vi "Edit Line.vi"(8 "error in (no error)":errorcluster, 10 "Line Name":string, 11 "object Refs":T1) -> (0 "error out":errorcluster, 1 "Change":bool)   [LabVIEW 2013, in "Modbus Module editor node.lvclass"]
uses:
  Modbus Module editor node.lvclass
  <vilib>/NI/DCAF/Tag Editor Core/Table API/Table Manager/object ref.ctl
  <vilib>/NI/DCAF/Tag Editor Core/Configuration Editor/Classes/Engine Parent/Engine Parent Editor Node.lvclass
  <vilib>/NI/DCAF/Tag Editor Core/Configuration Editor/Classes/Module editor node/module editor node.lvclass
  module/configuration/Modbus Module configuration.lvclass
  table line.ctl
  module/module channel/Modbus Module Channel.lvclass
  <vilib>/NI/Configuration Framework/serializable configuration/NISE_CEF_serializable configuration.lvclass/NISE_CEF_serializable configuration.ctl
  <vilib>/NI/Tag Bus/tag/tag descriptor.lvclass/tag descriptor.ctl
  <vilib>/Utility/LVClass/Get LV Class Name.vi
  <vilib>/NI/Configuration Framework/error generator/NISE_error generator.vi
  <vilib>/NI/Module Execution Interface/Engine Configuration/engine configuration.lvclass
  <vilib>/NI/Tag Bus/tag/tag descriptor.lvclass
  <vilib>/NI/Configuration Framework/serializable configuration/NISE_CEF_serializable configuration.lvclass
  <vilib>/NI/DCAF/Tag Editor Core/Table API/Table Manager/Table Manager.lvclass
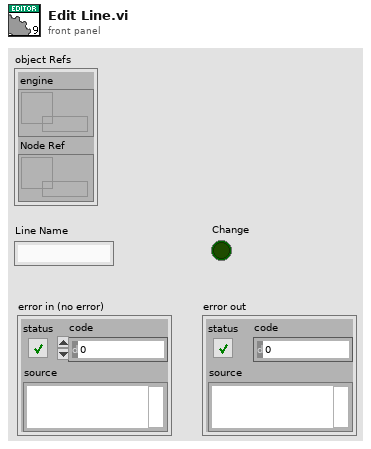
[diagram p1: front panel]
types:
  T1 = typedef "Table Manager.lvlib/Table Manager.lvclass/object ref.ctl" = cluster{"engine":refnum<data-value>, "Node Ref":refnum<data-value>}
  T2 = typedef "Modbus Module editor node.lvclass/table line.ctl" = cluster{"mbchan":refnum<class "Modbus Module Channel.lvclass">, "tag name":string}
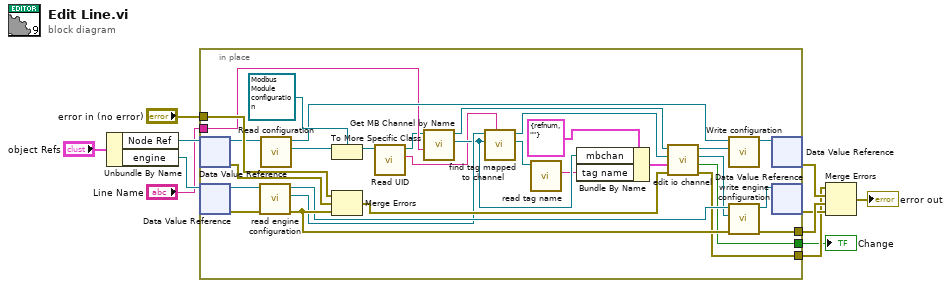
[diagram p0: block diagram]
diagram:
  n1 = Unbundle By Name("object Refs") -> ("Node Ref"=w4:refnum<data-value>, "engine"=w3:refnum<data-value>)
  n2 = in-place {
    in-place-border: [w33] -> w6
    in-place-border: "error in (no error)" -> [w41]
    in-place-border: [w35] -> w8
    in-place-border: "Line Name" -> [w22]
    in-place-border: [w12] -> w1
    n3 = in-place-dvr #1(w4) -> (w25:refnum<class "module editor node.lvclass">, w34:errorcluster)
    n4 = in-place-dvr #2(w3) -> (w40:refnum<class "Engine Parent Editor Node.lvclass">, w39:errorcluster)
    n5 = call <vilib>:"read engine configuration.vi"("error in"=w39, "Engine Parent Editor Node in"=w40) -> ("error out"=w37:errorcluster, "engine configuration"=w20:refnum<class "engine configuration.lvclass">, "Engine Parent Editor Node out"=w36:refnum<class "Engine Parent Editor Node.lvclass">)  [unwired: 7 in]
    n6 = call-dynamic "Read configuration.vi"("NISE_CEF_serializable node in"=w25) -> ("configuration"=w29:refnum<class "NISE_CEF_serializable configuration.lvclass">, "NISE_CEF_serializable node out"=w26:refnum<class "module editor node.lvclass">)  [unwired: 8 in, 1 out]
    n7 = To More Specific Class(target class=refnum<class "Modbus Module configuration.lvclass"> refnum ("Modbus Slave configuration in"), reference=w29) -> (specific class reference=w15:refnum<class "Modbus Module configuration.lvclass">)  [unwired: 1 in, 1 out]
    n8 = Merge Errors(w41, w34, w37) -> (w31:errorcluster)
    n9 = call <vilib>:"Read UID.vi"("configuration in"=w15) -> ("instance id"=w14:string, "configuration out"=w13:refnum<class "Modbus Module configuration.lvclass">)  [unwired: 8 in, 1 out]
    n10 = call "Get MB Channel by Name.vi"("Active Line Name"=w22, "Modbus Module configuration in"=w13) -> ("Modbus Module Channel.lvclass"=w18:refnum<class "Modbus Module Channel.lvclass">, "Modbus Module configuration out"=w21:refnum<class "Modbus Module configuration.lvclass">)  [unwired: 6 in, 2 out]
    n11 = call <vilib>:"find tag mapped to channel.vi"("owner"=w14, "channel"=w18, "engine configuration in"=w20) -> ("tag"=w17:refnum<class "tag descriptor.lvclass">, "engine configuration out"=w19:refnum<class "engine configuration.lvclass">)  [unwired: 6 in, 1 out]
    n12 = call <vilib>:"read tag name.vi"("system tag in"=w17) -> ("name"=w16:string)  [unwired: 8 in, 2 out]
    n13 = Bundle By Name(cluster=T2 {"mbchan"=refnum, "tag name"=""} ("line"), "mbchan"=w18, "tag name"=w16) -> (w23:T2)
    n14 = call "edit io channel.vi"("error in"=w31, "line"=w23, "engine configuration in"=w19, "tag bus configurable plugin module configuration in"=w21) -> ("error out"=w33:errorcluster, "Change"=w12:bool, "engine configuration"=w32:refnum<class "engine configuration.lvclass">, "tag bus configurable plugin module configuration out"=w27:refnum<class "Modbus Module configuration.lvclass">)  [unwired: 4 in]
    n15 = call-dynamic "Write configuration.vi"("configuration"=w27, "NISE_CEF_serializable node in"=w26) -> ("NISE_CEF_serializable node out"=w28:refnum<class "module editor node.lvclass">)  [unwired: 8 in, 1 out]
    n16 = call <vilib>:"write engine configuration.vi"("error in"=w37, "engine configuration"=w32, "Engine Parent Editor Node in"=w36) -> ("error out"=w35:errorcluster, "Engine Parent Editor Node out"=w38:refnum<class "Engine Parent Editor Node.lvclass">)  [unwired: 7 in]
    n17 = in-place-dvr #1(w28) -> (w9:errorcluster)  [unwired: 1 out]
    n18 = in-place-dvr #2(w38) -> (w7:errorcluster)  [unwired: 1 out]
  }
  "Change" <- w1
  n19 = Merge Errors(w6, w9, w8, w7) -> (→"error out":errorcluster)
